vi "Start.vi"(8 "error in (no error)":errorcluster, 11 "Scope PXI Base CFG in":refnum<class "Scope PXI Base CFG.lvclass">) -> (0 "error out":errorcluster, 3 "Scope PXI Base CFG out":refnum<class "Scope PXI Base CFG.lvclass">)   [LabVIEW 2023, in "Scope PXI Base CFG.lvclass"]
uses:
  Scope PXI Base CFG.lvclass
  Scope PXI Base CFG.lvclass/Scope PXI Base CFG.ctl
  <vilib>/Utility/error.llb/Error Cluster From Error Code.vi
  <vilib>/ErrorRing/Error Ring.xnode
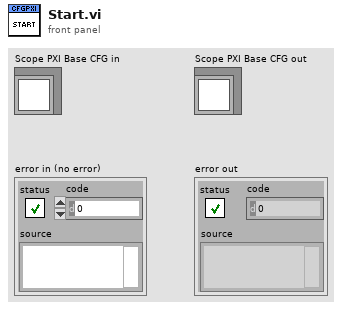
[diagram p1: front panel]
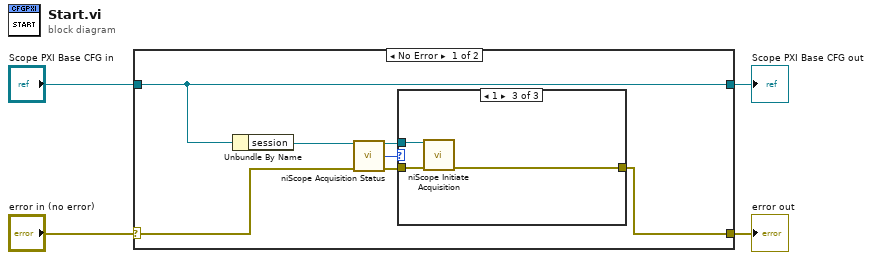
[diagram p0: block diagram]
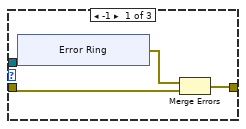
[diagram p2: hidden frame]
diagram:
  n1 = case shown="No Error" "error in (no error)" {
    selector: "error in (no error)" -> [w9 w25]
    tunnel: [w6 w25] -> w3
    tunnel: [w11 w24] -> w1
    tunnel: "Scope PXI Base CFG in" -> [w11 w24]
    frame No Error {
      n2 = Unbundle By Name(w11) -> ("session"=w10:refnum<k15>)
      n3 = call <instrlib>:"niScope Acquisition Status.vi"("instrument handle"=w10, "error in"=w9) -> ("instrument handle out"=w7:refnum<k15>, "acquisition status"=w5:i32, "error out"=w8:errorcluster)  [unwired: 11 in]
      n4 = case shown="1" w5 {
        tunnel: [w14 w20 w23] -> w6
        tunnel: w8 -> [w12 w20 w22]
        tunnel: w7 -> [_ _ w21]
        frame -1 {
          n5 = xnode "Error Ring"() -> ("error out"=w13:errorcluster)
          n6 = Merge Errors(w13, w12) -> (w14:errorcluster)
        }
        frame 0, Default {
        }
        frame 1 {
          n7 = call <instrlib>:"niScope Initiate Acquisition.vi"("instrument handle"=w21, "error in"=w22) -> ("error out"=w23:errorcluster)  [unwired: 12 in, 1 out]
        }
      }
    }
    frame Error {
    }
  }
  "error out" <- w3
  "Scope PXI Base CFG out" <- w1
